vi "Config Trig Edge.vi"(0 "VISA resource name":refnum<visa-resource-name>, 5 "Slope (0: RISE)":u16(ring) items=["RISE", "FALL", "BOTH"], 7 "Level (0)":dbl min=-100.0 max=100.0 step=0.10000000149011612 format="%.1f", 11 "error in (no error)":errorcluster) -> (4 "VISA resource name out":refnum<visa-resource-name>, 15 "error out":errorcluster)   [LabVIEW 2013, in "Yokogawa PZ4000.lvlib"]
doc: "This VI sends the Trigger Control command to the PZ4000.\nConfiguration Functions are Trigger Slope, and Level."
uses:
  Yokogawa PZ4000.lvlib
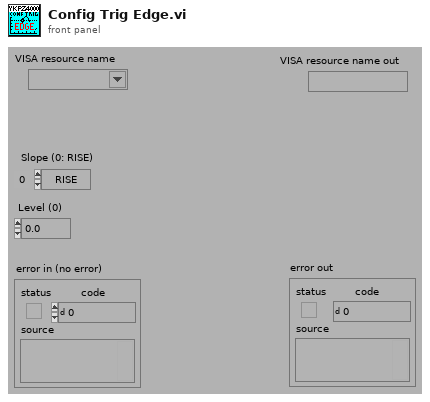
[diagram p1: front panel]
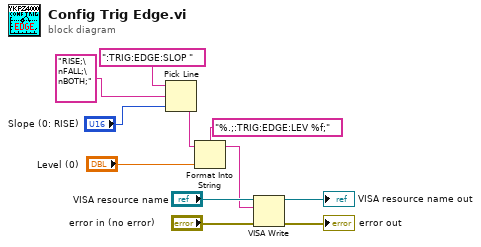
[diagram p0: block diagram]
diagram:
  n1 = Pick Line(string ("")=":TRIG:EDGE:SLOP ", multi-line string="RISE;\nFALL;\nBOTH;", line index="Slope (0: RISE)") -> (output string=w2:string)
  n2 = Format Into String(format string="%.;:TRIG:EDGE:LEV %f;", initial string=w2, "Level (0)") -> (resulting string=w1:string)  [unwired: 1 in, 1 out]
  n3 = VISA Write(VISA resource name="VISA resource name", write buffer=w1, error in (no error)="error in (no error)") -> (VISA resource name out=→"VISA resource name out":refnum<visa-resource-name>, error out=→"error out":errorcluster)  [unwired: 1 out]
